vi "stepperMotor.vi"() -> ()   [LabVIEW 2020]
uses:
  <vilib>/LabVIEW Interface for Arduino/Type Defs/Board Type.ctl
  <vilib>/LabVIEW Interface for Arduino/LabVIEW Interface for Arduino.lvlib
panel:
  in  "CCW - Pin Values 3":bool[](array[boolean])
  in  "CCW - Pin Values 2":bool[](array[boolean])
  in  "CCW - Pin Values 1":bool[](array[boolean])
  in  "CCW-Pin Values 0":bool[](array[boolean])
  in  "Clockwise":bool
  in  "Degrees":dbl
  in  "Pin Values 0":bool[](array[boolean])
  in  "Pin Values 3":bool[](array[boolean])
  in  "Pin Values 2":bool[](array[boolean])
  in  "Pin Values 1":bool[](array[boolean])
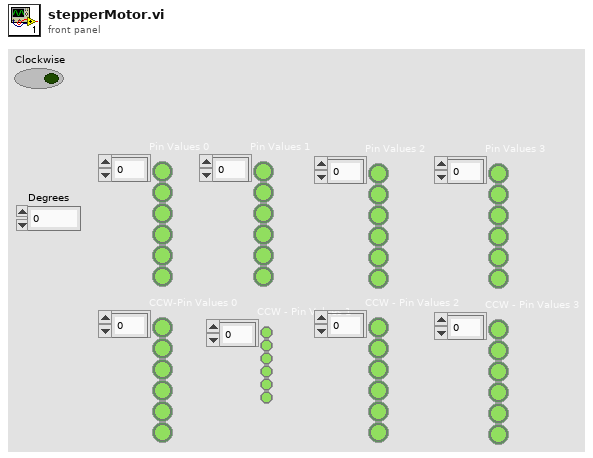
[diagram p1: front panel]
types:
  T1 = typedef "LabVIEW Interface for Arduino.lvlib/Board Type.ctl" = enum16{"Uno", "Dimuelanove w/Atmega 328", "Mega 2560"}
  T2 = typedef "LabVIEW Interface for Arduino.lvlib/Arduino Resource.ctl" = cluster{"VISA resource":refnum<visa-resource-name>, "Board Type":T1, "Connection Type":enum8{"USB / Serial"}, "Bytes Per Packet (15)":u8}
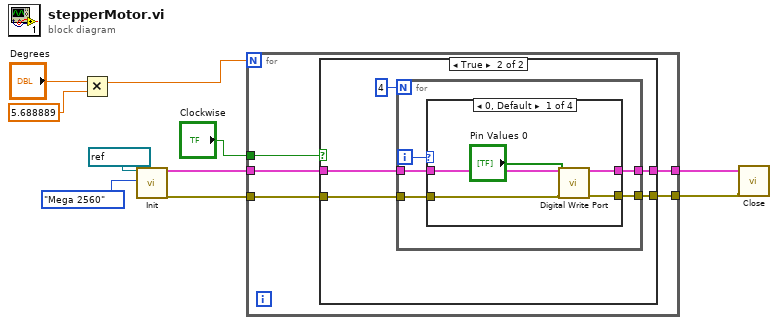
[diagram p0: block diagram]
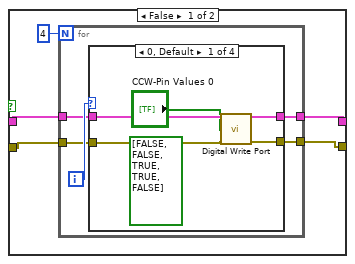
[diagram p2: hidden frame]
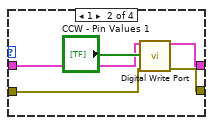
[diagram p3: hidden frame]
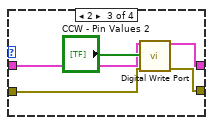
[diagram p4: hidden frame]
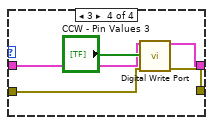
[diagram p5: hidden frame]
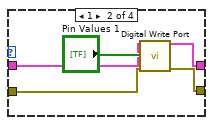
[diagram p6: hidden frame]
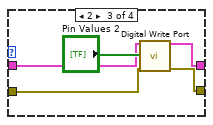
[diagram p7: hidden frame]
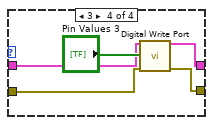
[diagram p8: hidden frame]
diagram:
  n1 = Multiply(x="Degrees", y=5.688889) -> (x*y=w3:dbl)
  n2 = call <vilib>:"Init.vi"("VISA resource"=refnum<visa-resource-name> "COM6", "Board Type (Uno)"=Board_Type."Mega 2560") -> ("Arduino Resource"=w10:T2, "error out"=w9:errorcluster)  [unwired: 16 in]
  n3 = for {
    N: w3 -> [_]
    tunnel: w10 -> [w15]
    tunnel: [w14] -> w1
    tunnel: w9 -> [w13]
    tunnel: [w12] -> w8
    tunnel: "Clockwise" -> [w11]
    n4 = case shown="True" w11 {
      tunnel: w15 -> [w17 w49]
      tunnel: [w19 w48] -> w14
      tunnel: w13 -> [w16 w47]
      tunnel: [w18 w46] -> w12
      frame False {
        n5 = for {
          N: 4 -> [_]
          tunnel: [w24] -> w19
          tunnel: [w23] -> w18
          tunnel: w17 -> [w22]
          tunnel: w16 -> [w21]
          i -> [w25]
          n6 = case shown="0, Default" w25 {
            tunnel: w22 -> [w28 w34 w39 w44]
            tunnel: [w27 w33 w38 w43] -> w24
            tunnel: w21 -> [w30 w32 w37 w42]
            tunnel: [w29 w31 w36 w41] -> w23
            frame 0, Default {
              (unwired) bool[] [FALSE, FALSE, TRUE, TRUE, FALSE] ("Pin Values")
              n7 = call <vilib>:"Digital Write Port.vi"("Arduino Resource"=w28, "Pin Values"="CCW-Pin Values 0", "error in"=w30) -> ("Arduino Resource"=w27:T2, "error out"=w29:errorcluster)  [unwired: 11 in]
            }
            frame 1 {
              n8 = call <vilib>:"Digital Write Port.vi"("Arduino Resource"=w34, "Pin Values"="CCW - Pin Values 1", "error in"=w32) -> ("Arduino Resource"=w33:T2, "error out"=w31:errorcluster)  [unwired: 11 in]
            }
            frame 2 {
              n9 = call <vilib>:"Digital Write Port.vi"("Arduino Resource"=w39, "Pin Values"="CCW - Pin Values 2", "error in"=w37) -> ("Arduino Resource"=w38:T2, "error out"=w36:errorcluster)  [unwired: 11 in]
            }
            frame 3 {
              n10 = call <vilib>:"Digital Write Port.vi"("Arduino Resource"=w44, "Pin Values"="CCW - Pin Values 3", "error in"=w42) -> ("Arduino Resource"=w43:T2, "error out"=w41:errorcluster)  [unwired: 11 in]
            }
          }
        }
      }
      frame True {
        n11 = for {
          N: 4 -> [_]
          tunnel: w49 -> [w54]
          tunnel: [w53] -> w48
          tunnel: w47 -> [w52]
          tunnel: [w51] -> w46
          i -> [w55]
          n12 = case shown="0, Default" w55 {
            tunnel: w54 -> [w59 w64 w69 w74]
            tunnel: [w58 w63 w68 w73] -> w53
            tunnel: w52 -> [w57 w62 w67 w72]
            tunnel: [w56 w61 w66 w71] -> w51
            frame 0, Default {
              n13 = call <vilib>:"Digital Write Port.vi"("Arduino Resource"=w59, "Pin Values"="Pin Values 0", "error in"=w57) -> ("Arduino Resource"=w58:T2, "error out"=w56:errorcluster)  [unwired: 11 in]
            }
            frame 1 {
              n14 = call <vilib>:"Digital Write Port.vi"("Arduino Resource"=w64, "Pin Values"="Pin Values 1", "error in"=w62) -> ("Arduino Resource"=w63:T2, "error out"=w61:errorcluster)  [unwired: 11 in]
            }
            frame 2 {
              n15 = call <vilib>:"Digital Write Port.vi"("Arduino Resource"=w69, "Pin Values"="Pin Values 2", "error in"=w67) -> ("Arduino Resource"=w68:T2, "error out"=w66:errorcluster)  [unwired: 11 in]
            }
            frame 3 {
              n16 = call <vilib>:"Digital Write Port.vi"("Arduino Resource"=w74, "Pin Values"="Pin Values 3", "error in"=w72) -> ("Arduino Resource"=w73:T2, "error out"=w71:errorcluster)  [unwired: 11 in]
            }
          }
        }
      }
    }
  }
  n17 = call <vilib>:"Close.vi"("Arduino Resource"=w1, "error in"=w8) -> ()  [unwired: 13 in, 1 out]
